vi "retrieveState.vi"(8 "error in (no error)":errorcluster, 11 "Model in":refnum<class "Model.lvclass">) -> (0 "error out":errorcluster, 2 "state":refnum<class "State.lvclass">, 3 "Model out":refnum<class "Model.lvclass">)   [LabVIEW 2013, in "Model.lvclass"]
uses:
  Model.lvclass
  State/State.lvclass
  Model.lvclass/Model.ctl
  IStateFactory/IStateFactory.lvclass
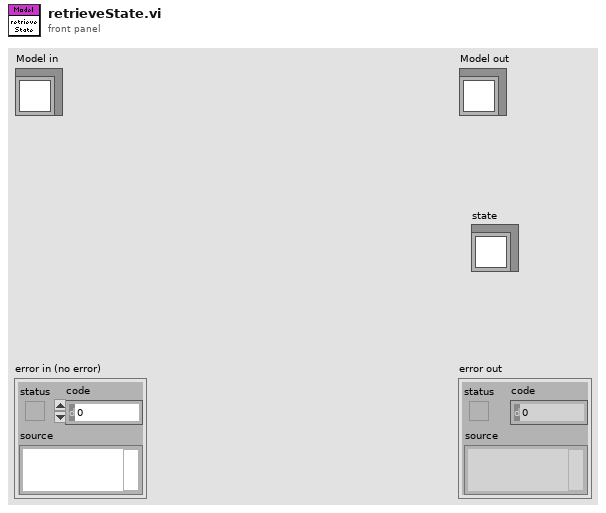
[diagram p1: front panel]
types:
  T1 = typedef "FAMTTypedefs.lvlib/StateSelector.ctl" = enum16{"EndingCycleState", "FaultState", "InteractiveSetpointState", "OffState", "StandbyState", "StoppedState"}
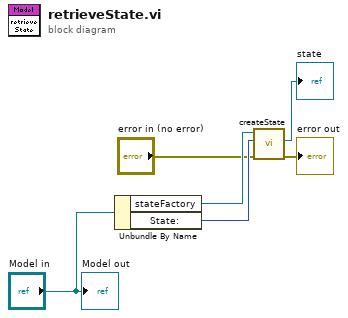
[diagram p0: block diagram]
diagram:
  n1 = Unbundle By Name("Model in") -> ("stateFactory"=w5:refnum<class "IStateFactory.lvclass">, "State:"=w4:T1)
  n2 = call-dynamic "createState.vi"("error in (no error)"="error in (no error)", "State:"=w4, "IStateFactory in"=w5) -> ("error out"=→"error out":errorcluster, "State.lvclass"=→"state":refnum<class "State.lvclass">)  [unwired: 6 in, 1 out]
  "Model out" <- "Model in"
